vi "RT_q2DCM (SubVI).vi"(11 "Quaternion":dbl[](array[numeric])=[0.0, 0.0, 0.0, 1.0]) -> (3 "DCM":dbl[][](array[numeric]))   [LabVIEW 2017]
panel:
  out "DCM line 3":dbl[](array[numeric])
  out "DCM line 2":dbl[](array[numeric])
  out "DCM line 1":dbl[](array[numeric])
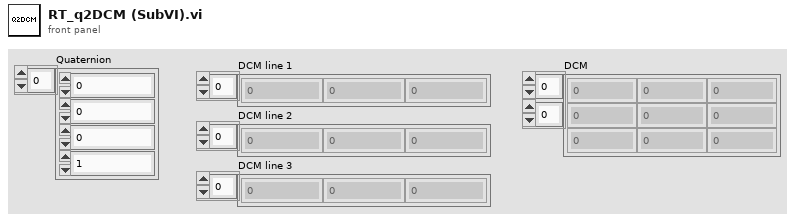
[diagram p1: front panel]
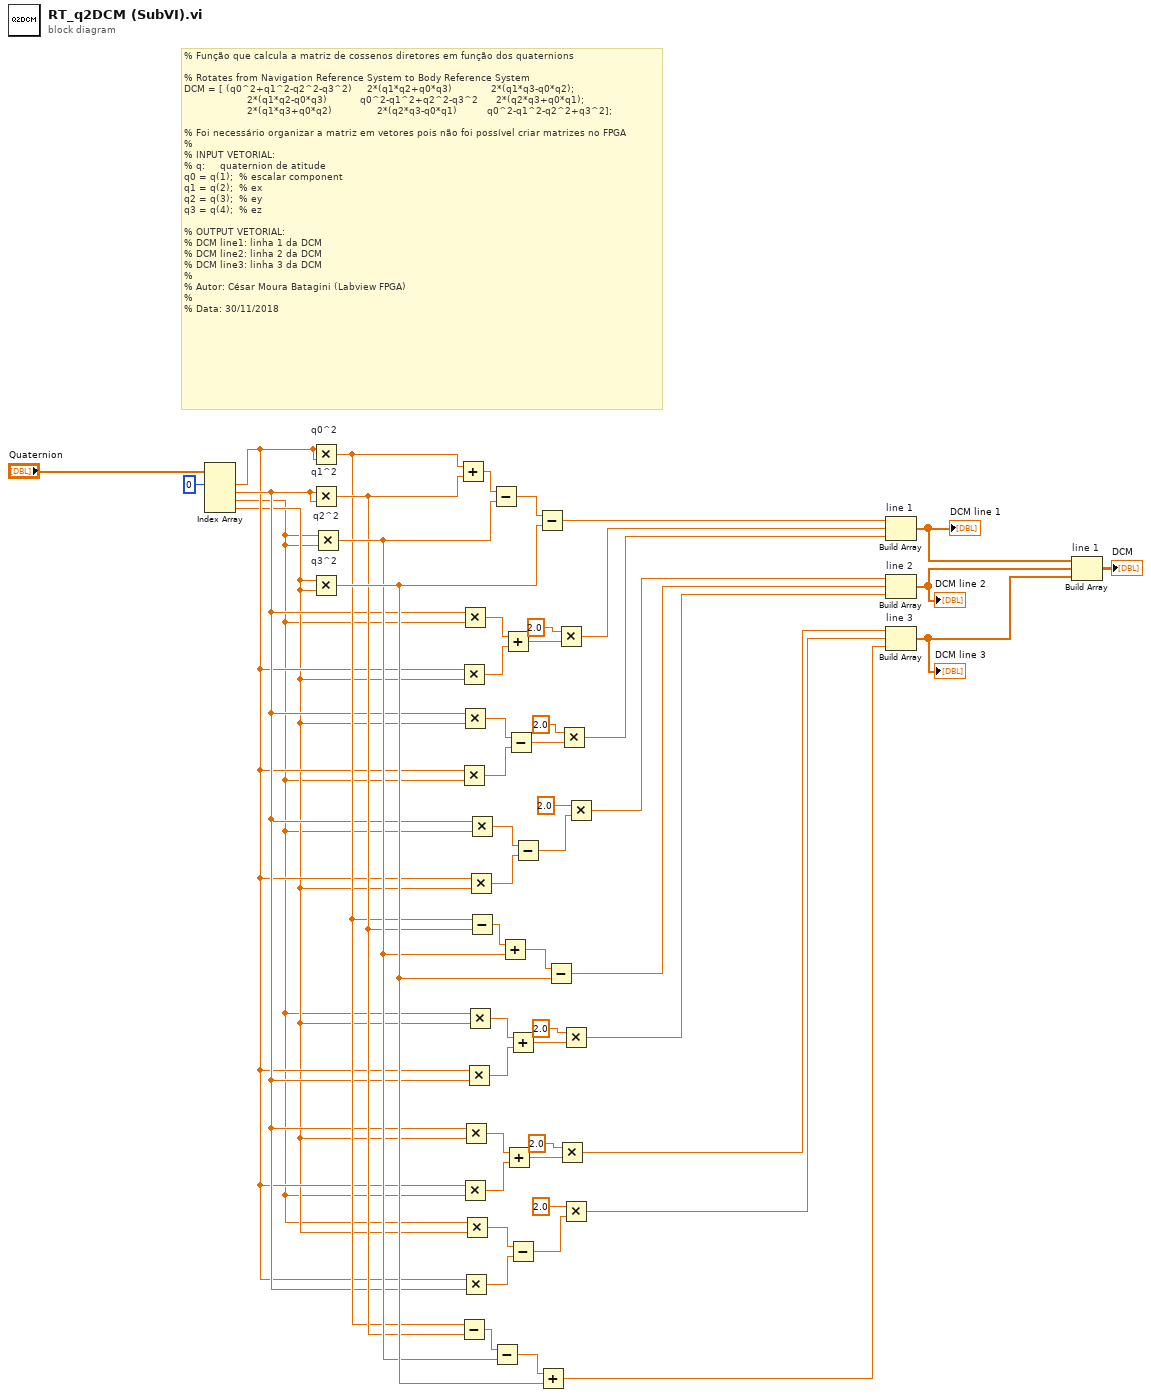
[diagram p0: block diagram]
diagram:
  # "% Função que calcula a matriz de cossenos diretores em função dos quaternions\n\n% Rotates from Navigation Reference System to Body Reference System\nDCM = [ (q0^2+q1^2-q2^2-q3^2)     2*(q1*q2+q0*q3)             2*(q1*q3-q0*q2);\n                     2*(q1*q2-q0*q3)           q0^2-q1^2+q2^2-q3^2      2*(q2*q3+q0*q1);\n                     2*(q1*q3+q0*q2)               2*(q2*q3-q0*q1)          q0^2-q1^2-q2^2+q3^2];\n\n% Foi necessário organizar a matriz em vetores pois não foi possível criar matrizes no FPGA\n%\n% INPUT VETORIAL: \n% q:     quaternion de atitude   \nq0 = q(1);  % escalar component\nq1 = q(2);  % ex\nq2 = q(3);  % ey\nq3 = q(4);  % ez\n\n% OUTPUT VETORIAL:\n% DCM line1: linha 1 da DCM\n% DCM line2: linha 2 da DCM\n% DCM line3: linha 3 da DCM\n%\n% Autor: César Moura Batagini (Labview FPGA)\n%             \n% Data: 30/11/2018"
  n1 = Index Array(array="Quaternion", index #1=0 ("index")) -> (element #1=w48:dbl, element #2=w49:dbl, element #3=w46:dbl, element #4=w47:dbl)  [unwired: 3 in]
  n2 = Multiply "q0^2"(x=w48, y=w48) -> (x*y=w50:dbl)
  n3 = Multiply "q1^2"(x=w49, y=w49) -> (x*y=w51:dbl)
  n4 = Multiply "q3^2"(x=w47, y=w47) -> (x*y=w53:dbl)
  n5 = Multiply "q2^2"(x=w46, y=w46) -> (x*y=w52:dbl)
  n6 = Add(x=w50, y=w51) -> (x+y=w15:dbl)
  n7 = Multiply(x=w48, y=w47) -> (x*y=w19:dbl)
  n8 = Multiply(x=w48, y=w46) -> (x*y=w27:dbl)
  n9 = Subtract(x=w50, y=w51) -> (x-y=w43:dbl)
  n10 = Multiply(x=w49, y=w46) -> (x*y=w18:dbl)
  n11 = Multiply(x=w49, y=w47) -> (x*y=w26:dbl)
  n12 = Multiply(x=w48, y=w46) -> (x*y=w37:dbl)
  n13 = Multiply(x=w49, y=w47) -> (x*y=w36:dbl)
  n14 = Multiply(x=w48, y=w49) -> (x*y=w41:dbl)
  n15 = Multiply(x=w46, y=w47) -> (x*y=w40:dbl)
  n16 = Multiply(x=w48, y=w49) -> (x*y=w32:dbl)
  n17 = Multiply(x=w46, y=w47) -> (x*y=w33:dbl)
  n18 = Multiply(x=w48, y=w47) -> (x*y=w22:dbl)
  n19 = Multiply(x=w49, y=w46) -> (x*y=w23:dbl)
  n20 = Subtract(x=w50, y=w51) -> (x-y=w30:dbl)
  n21 = Subtract(x=w15, y=w52) -> (x-y=w16:dbl)
  n22 = Subtract(x=w43, y=w52) -> (x-y=w44:dbl)
  n23 = Add(x=w30, y=w52) -> (x+y=w29:dbl)
  n24 = Add(x=w18, y=w19) -> (x+y=w20:dbl)
  n25 = Add(x=w36, y=w37) -> (x+y=w38:dbl)
  n26 = Subtract(x=w26, y=w27) -> (x-y=w28:dbl)
  n27 = Add(x=w33, y=w32) -> (x+y=w31:dbl)
  n28 = Subtract(x=w40, y=w41) -> (x-y=w42:dbl)
  n29 = Subtract(x=w23, y=w22) -> (x-y=w21:dbl)
  n30 = Subtract(x=w16, y=w53) -> (x-y=w12:dbl)
  n31 = Add(x=w44, y=w53) -> (x+y=w45:dbl)
  n32 = Subtract(x=w29, y=w53) -> (x-y=w8:dbl)
  n33 = Multiply(x=sgl 2.0, y=w20) -> (x*y=w11:dbl)
  n34 = Multiply(x=sgl 2.0, y=w38) -> (x*y=w6:dbl)
  n35 = Multiply(x=sgl 2.0, y=w28) -> (x*y=w10:dbl)
  n36 = Multiply(x=sgl 2.0, y=w31) -> (x*y=w7:dbl)
  n37 = Multiply(x=sgl 2.0, y=w42) -> (x*y=w5:dbl)
  n38 = Multiply(x=sgl 2.0, y=w21) -> (x*y=w9:dbl)
  n39 = Build Array "line 1"(w12, w11, w10) -> (w4:dbl[])
  "DCM line 1" <- w4
  n40 = Build Array "line 2"(w9, w8, w7) -> (w3:dbl[])
  "DCM line 2" <- w3
  n41 = Build Array "line 3"(w6, w5, w45) -> (w2:dbl[])
  "DCM line 3" <- w2
  n42 = Build Array "line 1"(w4, w3, w2) -> (→"DCM":dbl[][])
